vi "SSC DCPower Finish Waveform Acquisition.vi"(0 "DCPower SSC in":T3[](array[typedef]), 1 "Settings":T1 {"Previous Settings"."Triggers:Measure Trigger:Trigger Type" items=["Digital Edge"=1014, "Software Edge"=1015, "None"=1012]; "Previous Settings"."Measurement:Advanced:Measure When" items=["Automatically after Source Complete"=1025, "On Demand"=1026, "On Measure Trigger"=1027]; "Previous Settings"."Measurement:Aperture Time" format="%#_6p"; "Previous Settings"."Measurement:Aperture Time Units" items=["Seconds"=1028, "Power Line Cycles"=1029]}, 5 "Fetch Waveform Length (s)":dbl, 11 "error in":errorcluster) -> (4 "DCPower SSC out":T3[](array[typedef]), 6 "Voltage Waveforms":waveform(dbl)[](graph), 8 "Current Waveforms":waveform(dbl)[](graph), 15 "error out":errorcluster)   [LabVIEW 2020]
doc: "This VI reconfigures the SMU to the previous settings and outputs the samples captured during waveform acquisition."
uses:
  SSC DCPower.ctl
  SSC DCPower Waveform Acquisition Saved Settings.ctl
  SSC DCPower Waveform Acquisition Saved Setting.ctl
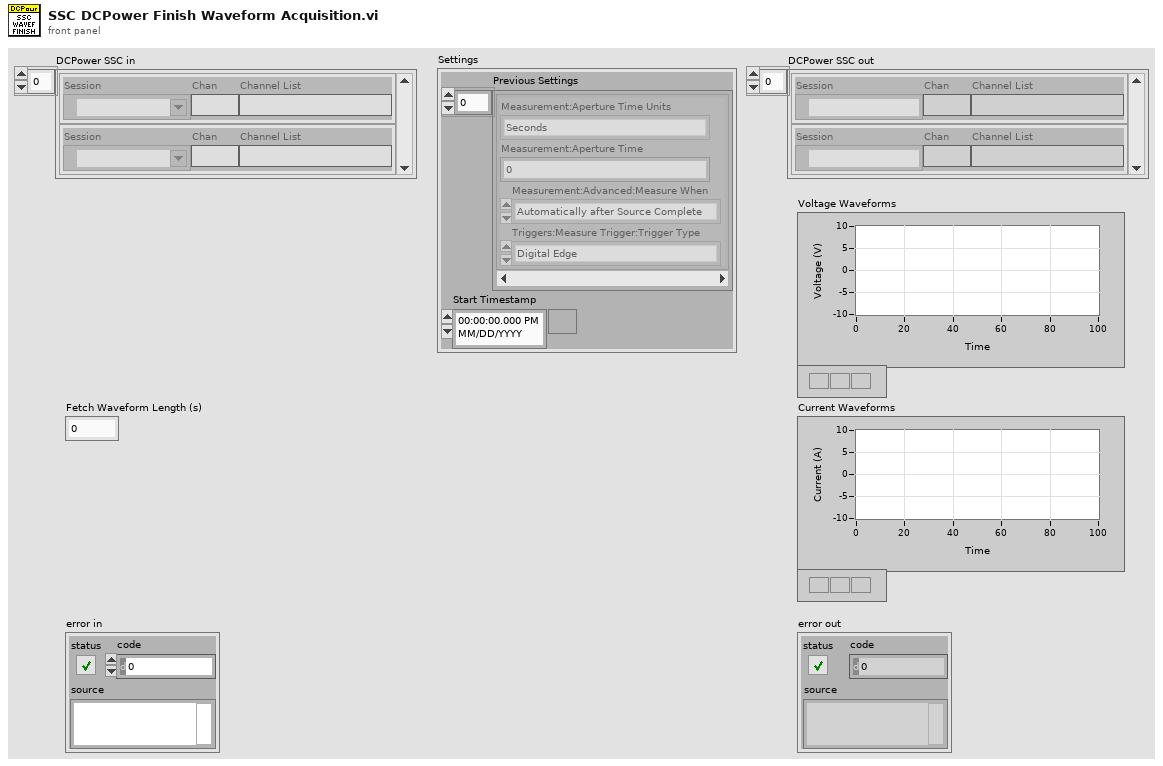
[diagram p1: front panel]
types:
  T1 = typedef "SSC DCPower Waveform Acquisition Saved Settings.ctl" = cluster{"Previous Settings":T2[], "Start Timestamp":timestamp}
  T2 = typedef "SSC DCPower Waveform Acquisition Saved Setting.ctl" = cluster{"Measurement:Aperture Time Units":i32, "Measurement:Aperture Time":dbl, "Measurement:Advanced:Measure When":i32, "Triggers:Measure Trigger:Trigger Type":i32}
  T3 = typedef "SSC DCPower.ctl" = cluster{"Session":refnum<k15>, "Chan":string, "Channel List":string}
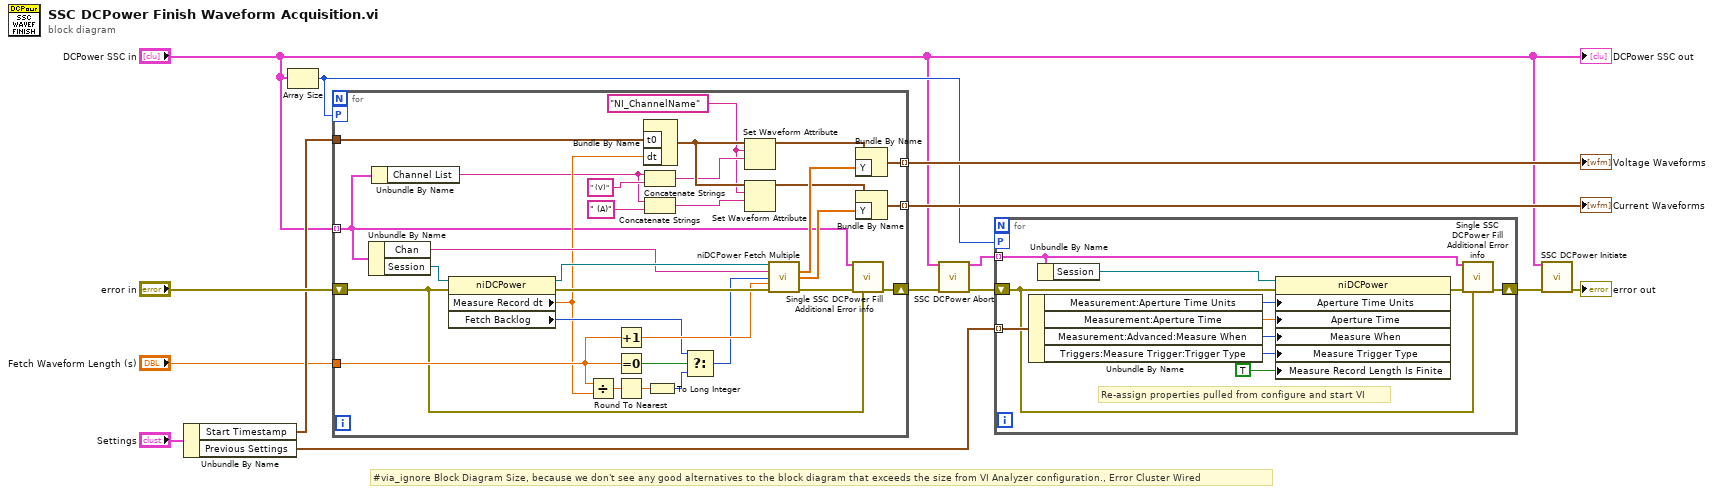
[diagram p0: block diagram]
diagram:
  # "#via_ignore Block Diagram Size, because we don't see any good alternatives to the block diagram that exceeds the size from VI Analyzer configuration., Error Cluster Wired"
  n1 = Unbundle By Name("Settings") -> ("Start Timestamp"=w9:timestamp, "Previous Settings"=w11:T2[])
  n2 = Array Size(array="DCPower SSC in") -> (size(s)=w5:i32)
  n3 = for {
    tunnel: "DCPower SSC in" -> [w16] mode=indexing
    workers-P: w5 -> [_]
    tunnel: [w44] -> w13 mode=indexing
    tunnel: [w43] -> w14 mode=indexing
    tunnel: w9 -> [w42]
    shift-right: [w25] -> w2
    shift-left: "error in" -> [w24]
    tunnel: "Fetch Waveform Length (s)" -> [w30]
    w17 = "NI_ChannelName"
    n4 = Unbundle By Name(w16) -> ("Chan"=w39:string, "Session"=w41:refnum<k15>)
    n5 = Unbundle By Name(w16) -> ("Channel List"=w15:string)
    n6 = property class="niDCPower"(reference=w41, error in=w24) -> (reference out=w40:refnum<k15>, error out=w35:errorcluster, "Measure Record dt"=w29:dbl, "Fetch Backlog"=w32:i32)
    n7 = Divide(x=w30, y=w29) -> (x/y=w28:dbl)
    n8 = Increment(x=w30) -> (x+1=w34:dbl)
    n9 = Equal To 0?(x=w30) -> (x = 0?=w33:bool)
    n10 = Round To Nearest(number=w28) -> (nearest integer value=w27:dbl)
    n11 = Bundle By Name("t0"=w42, "dt"=w29) -> (w37:waveform(dbl))  [unwired: 1 in]
    n12 = Concatenate Strings(w15, " (V)") -> (w21:string)
    n13 = Concatenate Strings(w15, " (A)") -> (w18:string)
    n14 = To Long Integer(number=w27) -> (32bit integer=w26:i32)
    n15 = Select(t=w32, s=w33, f=w26) -> (s? t:f=w31:i32)
    n16 = Set Waveform Attribute(5:w21, 6:w17, 7:w37) -> (3:w23:waveform(dbl))  [unwired: 1 in, 2 out]
    n17 = Set Waveform Attribute(5:w18, 6:w17, 7:w37) -> (3:w22:waveform(dbl))  [unwired: 1 in, 2 out]
    n18 = call <instrlib>:"niDCPower Fetch Multiple.vi"("instrument handle"=w40, "channel name"=w39, "count (1)"=w31, "timeout (sec)"=w34, "error in (no error)"=w35) -> ("voltage measurements"=w38:dbl[], "current measurements"=w36:dbl[], "error out"=w45:errorcluster)  [unwired: 5 in, 3 out]
    n19 = call "Single SSC DCPower Fill Additional Error info.vi"("DCPower SSC in"=w16, "error in"=w45, "previous error in"=w24) -> ("error out"=w25:errorcluster)  [unwired: 12 in]
    n20 = Bundle By Name(cluster=w23, "Y"=w38) -> (w44:waveform(dbl))
    n21 = Bundle By Name(cluster=w22, "Y"=w36) -> (w43:waveform(dbl))
  }
  "Voltage Waveforms" <- w13
  "Current Waveforms" <- w14
  n22 = call "SSC DCPower Abort.vi"("DCPower SSC in"="DCPower SSC in", "error in"=w2) -> ("DCPower SSC out"=w6:T3[], "error out"=w7:errorcluster)  [unwired: 12 in]
  n23 = for {
    tunnel: w6 -> [w47] mode=indexing
    workers-P: w5 -> [_]
    tunnel: w11 -> [w55] mode=indexing
    shift-right: [w48] -> w8
    shift-left: w7 -> [w46]
    # "Re-assign properties pulled from configure and start VI"
    n24 = Unbundle By Name(w55) -> ("Measurement:Aperture Time Units"=w53:i32, "Measurement:Aperture Time"=w52:dbl, "Measurement:Advanced:Measure When"=w51:i32, "Triggers:Measure Trigger:Trigger Type"=w50:i32)
    n25 = Unbundle By Name(w47) -> ("Session"=w54:refnum<k15>)
    n26 = property class="niDCPower"(reference=w54, error in=w46, "Aperture Time Units"=w53, "Aperture Time"=w52, "Measure When"=w51, "Measure Trigger Type"=w50, "Measure Record Length Is Finite"=TRUE ("Measurement:Measure Record Length Is Finite")) -> (error out=w56:errorcluster)  [unwired: 1 out]
    n27 = call "Single SSC DCPower Fill Additional Error info.vi"("DCPower SSC in"=w47, "error in"=w56, "previous error in"=w46) -> ("error out"=w48:errorcluster)  [unwired: 12 in]
  }
  n28 = call "SSC DCPower Initiate.vi"("DCPower SSC in"="DCPower SSC in", "error in"=w8) -> ("error out"=→"error out":errorcluster)  [unwired: 12 in, 1 out]
  "DCPower SSC out" <- "DCPower SSC in"
